vi "Start Configuration.vi"(6 "Ref Lvl Auto":bool, 8 "error in (no error)":errorcluster, 9 "Cluster de Dados":T1={"Limite de Temperatura"=27.0, "Temperatura"=25.0, "Corrente Inicial (mA)"=0.0, "Corrente Limite (mA)"=300, "Resolution"=enum."Normal", "Centro do Pico do espectro (nm)"=1550.0, "Valor de Span (nm)"=100.0, "Laser Led Select (Laser)"=enum."Laser"} {"Valor de Span (nm)" format="%.2f"; "Centro do Pico do espectro (nm)" format="%.2f"; "Corrente Inicial (mA)" min=0.0 step=1.0; "Temperatura" min=-100.0 max=199.9 step=0.1; "Limite de Temperatura" min=-100.0 max=199.9 step=0.1}, 10 "GPIB Espectrometro":refnum<visa-resource-name>="GPIB0::1::INSTR", 11 "GPIB Controlador Laser Diodo":refnum<visa-resource-name>="GPIB0::1::INSTR") -> (0 "error out":errorcluster, 2 "Spectrometer out":refnum<visa-resource-name>, 3 "Controller out":refnum<visa-resource-name>)   [LabVIEW 2018]
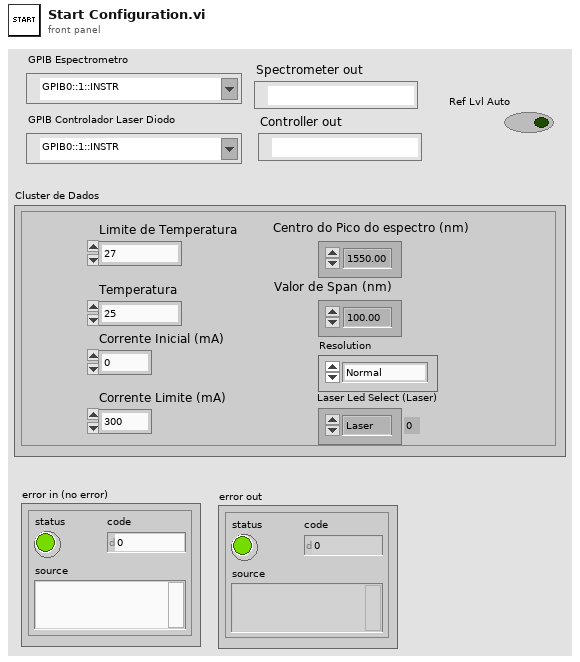
[diagram p1: front panel]
types:
  T1 = cluster{"Limite de Temperatura":dbl, "Temperatura":dbl, "Corrente Inicial (mA)":dbl, "Corrente Limite (mA)":i32, "Resolution":enum16{"Normal", "High"}, "Centro do Pico do espectro (nm)":dbl, "Valor de Span (nm)":dbl, "Laser Led Select (Laser)":enum16{"Laser", "Led"}}
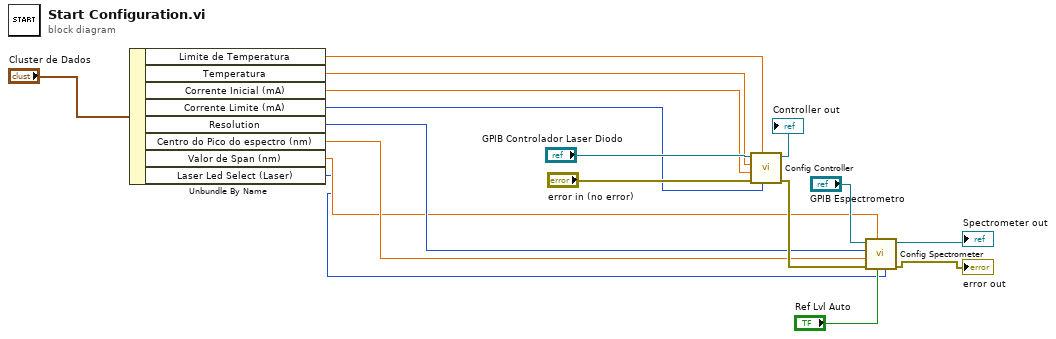
[diagram p0: block diagram]
diagram:
  n1 = Unbundle By Name("Cluster de Dados") -> ("Limite de Temperatura"=w12:dbl, "Temperatura"=w11:dbl, "Corrente Inicial (mA)"=w9:dbl, "Corrente Limite (mA)"=w10:i32, "Resolution"=w8:enum16{"Normal", "High"}, "Centro do Pico do espectro (nm)"=w7:dbl, "Valor de Span (nm)"=w6:dbl, "Laser Led Select (Laser)"=w1:enum16{"Laser", "Led"})
  n2 = call "Config Controller.vi"("Corrente Limite (mA)"=w10, "Limite de Temperatura"=w12, "error in (no error)"="error in (no error)", "Corrente Inicial (mA)"=w9, "Temperatura"=w11, "VISA Refnum in"="GPIB Controlador Laser Diodo") -> ("error out"=w14:errorcluster, "VISA Refnum out"=→"Controller out":refnum<visa-resource-name>)  [unwired: 4 in]
  n3 = call "Config Spectrometer.vi"("Laser Led Select (Laser)"=w1, "Ref Lvl Auto"="Ref Lvl Auto", "Valor de Span (nm)"=w6, "error in (no error)"=w14, "Centro do Pico do espectro (nm)"=w7, "Resolution"=w8, "VISA Refnum in"="GPIB Espectrometro") -> ("error out"=→"error out":errorcluster, "VISA Refnum out"=→"Spectrometer out":refnum<visa-resource-name>)  [unwired: 3 in]
